vi "Cholesky Decomposition.vi"(1 "n":i32, 2 "m":i32, 3 "A":sgl[](array[numeric])) -> (0 "L":sgl[](array[numeric]))   [LabVIEW 2020]
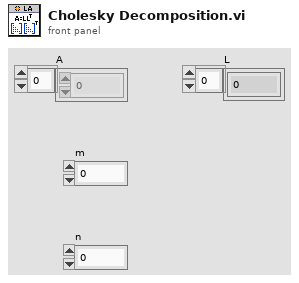
[diagram p1: front panel]
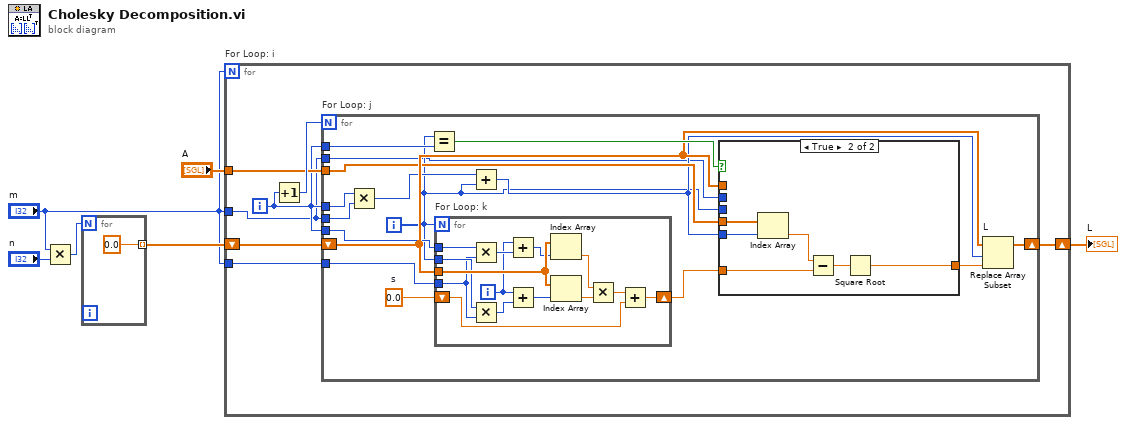
[diagram p0: block diagram]
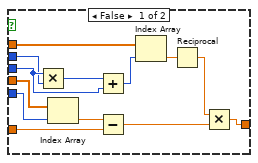
[diagram p2: hidden frame]
diagram:
  n1 = Multiply(x="m", y="n") -> (x*y=w1:i32)
  n2 = for {
    N: w1 -> [_]
    tunnel: [sgl 0.0] -> w4 mode=indexing
  }
  n3 = for "For Loop: i" {
    N: "m" -> [_]
    shift-right: [w12] -> w6
    shift-left: w4 -> [w14]
    tunnel: "A" -> [w11]
    tunnel: "m" -> [w9]
    tunnel: "m" -> [w8]
    i -> [w10]
    n4 = Increment(x=w10) -> (x+1=w13:i32)
    n5 = for "For Loop: j" {
      N: w13 -> [_]
      tunnel: w10 -> [w24]
      shift-right: [w26] -> w12
      shift-left: w14 -> [w25]
      tunnel: w10 -> [w23]
      tunnel: w11 -> [w21]
      tunnel: w10 -> [w19]
      tunnel: w9 -> [w17]
      tunnel: w9 -> [w16]
      tunnel: w8 -> [w15]
      i -> [w18]
      w29 = sgl 0.0  # s
      n6 = Multiply(x=w23, y=w17) -> (x*y=w22:i32)
      n7 = Equal?(x=w18, y=w24) -> (x = y?=w30:bool)
      n8 = for "For Loop: k" {
        N: w18 -> [_]
        tunnel: w25 -> [w62]
        shift-right: [w58] -> w28
        shift-left: w29 -> [w59]
        tunnel: w19 -> [w57]
        tunnel: w18 -> [w52]
        tunnel: w15 -> [w50]
        i -> [w51]
        n9 = Multiply(x=w57, y=w50) -> (x*y=w56:i32)
        n10 = Multiply(x=w52, y=w50) -> (x*y=w54:i32)
        n11 = Add(x=w51, y=w56) -> (x+y=w55:i32)
        n12 = Add(x=w51, y=w54) -> (x+y=w53:i32)
        n13 = Index Array(array=w62, index=w55) -> (element=w63:sgl)
        n14 = Index Array(array=w62, index=w53) -> (element=w61:sgl)
        n15 = Multiply(x=w63, y=w61) -> (x*y=w60:sgl)
        n16 = Add(x=w60, y=w59) -> (x+y=w58:sgl)
      }
      n17 = Add(x=w22, y=w18) -> (x+y=w20:i32)
      n18 = case shown="True" w30 {
        tunnel: w28 -> [w41 w49]
        tunnel: [w40 w47] -> w27
        tunnel: w25 -> [w43 _]
        tunnel: w21 -> [w37 w46]
        tunnel: w20 -> [w36 w45]
        tunnel: w18 -> [w33 _]
        tunnel: w16 -> [w31 _]
        frame False {
          n19 = Multiply(x=w33, y=w31) -> (x*y=w34:i32)
          n20 = Index Array(array=w37, index=w36) -> (element=w35:sgl)
          n21 = Add(x=w34, y=w33) -> (x+y=w32:i32)
          n22 = Subtract(x=w35, y=w41) -> (x-y=w38:sgl)
          n23 = Index Array(array=w43, index=w32) -> (element=w42:sgl)
          n24 = Reciprocal(x=w42) -> (1/x=w39:sgl)
          n25 = Multiply(x=w39, y=w38) -> (x*y=w40:sgl)
        }
        frame True {
          n26 = Index Array(array=w46, index=w45) -> (element=w44:sgl)
          n27 = Subtract(x=w44, y=w49) -> (x-y=w48:sgl)
          n28 = Square Root(x=w48) -> (sqrt(x)=w47:sgl)
        }
      }
      n29 = Replace Array Subset "L"(array=w25, new element=w27, index=w20) -> (w26:sgl[])
    }
  }
  "L" <- w6
